vi "Pack Four 16-bit to 64-bit (Single Tick).vi"(7 "Swap I16 Numbers":bool=TRUE, 8 "Input Valid":bool=TRUE, 11 "Input data":cluster{"d0":i16, "d1":i16, "d2":i16, "d3":i16}) -> (0 "Output Valid":bool=TRUE, 3 "Output Data":u64)   [LabVIEW 2011]
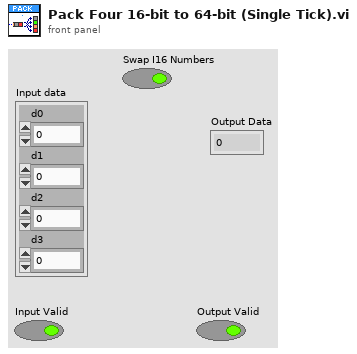
[diagram p1: front panel]
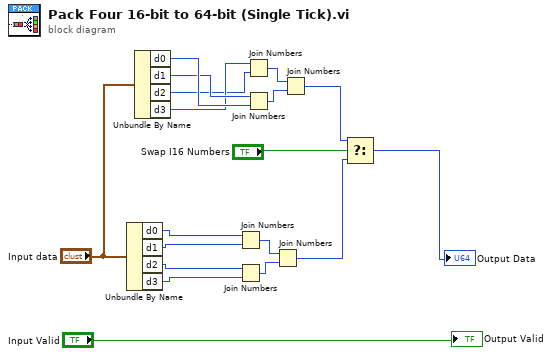
[diagram p0: block diagram]
diagram:
  n1 = Unbundle By Name("Input data") -> ("d0"=w16:i16, "d1"=w15:i16, "d2"=w14:i16, "d3"=w13:i16)
  n2 = Unbundle By Name("Input data") -> ("d0"=w5:i16, "d1"=w4:i16, "d2"=w1:i16, "d3"=w2:i16)
  n3 = Join Numbers(hi=w16, lo=w15) -> ((hi.lo)=w17:u32)
  n4 = Join Numbers(hi=w14, lo=w13) -> ((hi.lo)=w18:u32)
  n5 = Join Numbers(hi=w2, lo=w1) -> ((hi.lo)=w8:u32)
  n6 = Join Numbers(hi=w4, lo=w5) -> ((hi.lo)=w7:u32)
  n7 = Join Numbers(hi=w17, lo=w18) -> ((hi.lo)=w10:u64)
  n8 = Join Numbers(hi=w8, lo=w7) -> ((hi.lo)=w3:u64)
  n9 = Select(t=w3, s="Swap I16 Numbers", f=w10) -> (s? t:f=→"Output Data":u64)
  "Output Valid" <- "Input Valid"
